vi "Enqueuer.vi"(8 "error in (no error)":errorcluster, 11 "RemoteCommandable in":refnum<class "RemoteCommandable.lvclass">) -> (0 "error out":errorcluster, 2 "EnQr":refnum<class "Message Enqueuer.lvclass">, 3 "RemoteCommandable out":refnum<class "RemoteCommandable.lvclass">)   [LabVIEW 2020, in "Volatus.lvlib" / "RemoteCommandable.lvclass"]
uses:
  RemoteCommandable.lvclass
  <vilib>/ActorFramework/Message Enqueuer/Message Enqueuer.lvclass
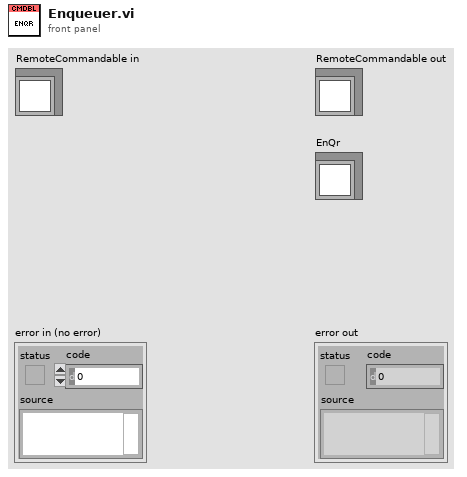
[diagram p1: front panel]
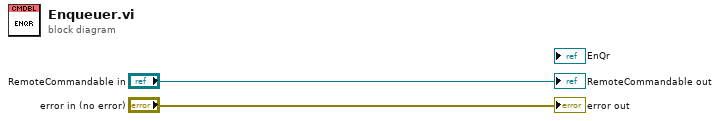
[diagram p0: block diagram]
diagram:
  "error out" <- "error in (no error)"
  "RemoteCommandable out" <- "RemoteCommandable in"
